vi "song playing.vi"() -> ()   [LabVIEW 2020]
panel:
  in  "Path":path
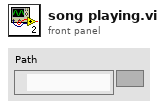
[diagram p1: front panel]
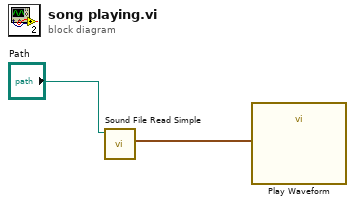
[diagram p0: block diagram]
diagram:
  n1 = call <vilib>:"Sound File Read Simple.vi"("path"="Path") -> ("data"=w1:waveform(dbl)[])  [unwired: 7 in, 3 out]
  n2 = call "Play Waveform"("Data"=w1) -> ()  [unwired: 18 in, 1 out]
